vi "CRC16_Modbus.vi"(1 "需要校验的数据":string) -> (0 "String+CRC16":string)   [LabVIEW 2015]
panel:
  out "CRCLo":u8 format="%x"
  out "CRCHI":u8 format="%x"
  out "CRC16Modbus":string
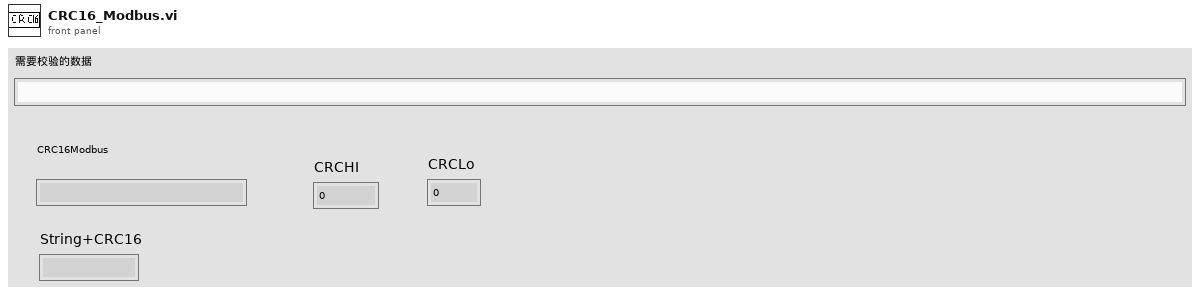
[diagram p1: front panel]
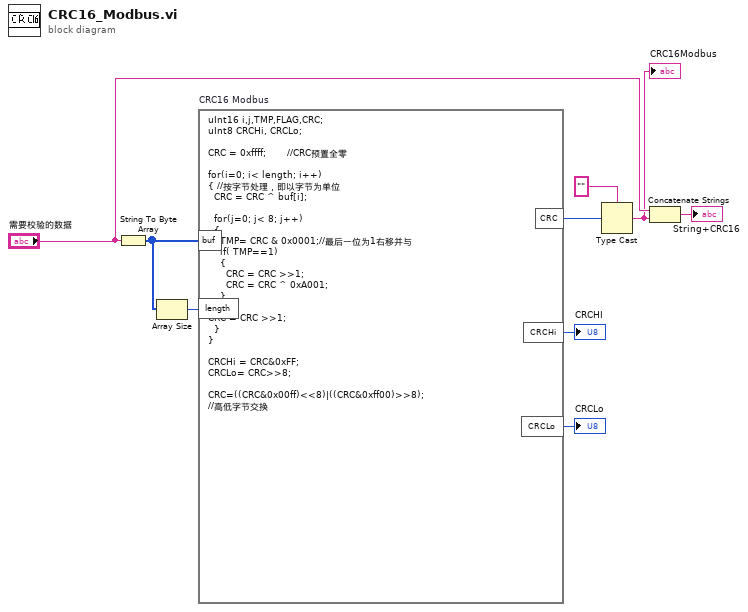
[diagram p0: block diagram]
diagram:
  n1 = String To Byte Array(string="需要校验的数据") -> (unsigned byte array=w9:u8[])
  n2 = Array Size(array=w9) -> (size(s)=w8:i32)
  n3 = formula code="uInt16 i,j,TMP,FLAG,CRC;\nuInt8 CRCHi, CRCLo;\n\nCRC = 0xffff;       //CRC预置全零\n\nfor(i=0; i< length; i++)\n{ //按字节处理，即以字节为单位\n  CRC = CRC ^ buf[i];\n\n  for(j=0; j< 8; j++)\n  { \n    TMP= CRC & 0x0001;//最后一位为1右移并与\n    if( TMP==1)\n    { \n      CRC = CRC >>1;\n      CRC = CRC ^ 0xA001;\n    }\nelse\nCRC = CRC >>1;\n  } \n}\n\nCRCHi = CRC&0xFF;\nCRCLo= CRC>>8;\n\nCRC=((CRC&0x00ff)<<8)|((CRC&0xff00)>>8);\n//高低字节交换" "CRC16 Modbus"("buf"=w9, "length"=w8) -> ("CRC"=w6:u16, "CRCHi"=→"CRCHI":u8, "CRCLo"=→"CRCLo":u8)
  n4 = Type Cast(type="" ("类型"), x=w6) -> (*(type *) &x=w2:string)
  "CRC16Modbus" <- w2
  n5 = Concatenate Strings("需要校验的数据", w2) -> (→"String+CRC16":string)
